vi "GetLineage.vi"(8 "error in (no error)":errorcluster, 11 "SMO in":refnum<class "SMO.lvclass">) -> (0 "error out":errorcluster, 2 "Lineage":string[](array[string]), 3 "SMO out":refnum<class "SMO.lvclass">)   [LabVIEW 2021, in "smo.lvlib" / "SMO.lvclass"]
uses:
  SMO.lvclass
  Support/Attribute.Owner/Attribute.Owner.lvclass
  SMO.lvclass/SMO.ctl
  Support/Attribute.Owner/Attribute.Owner.lvclass/Attribute.Owner.ctl
  ReftoDVR--SMO.vi
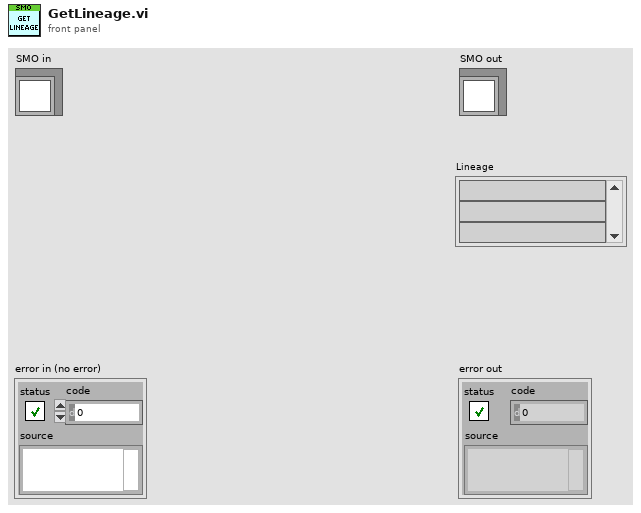
[diagram p1: front panel]
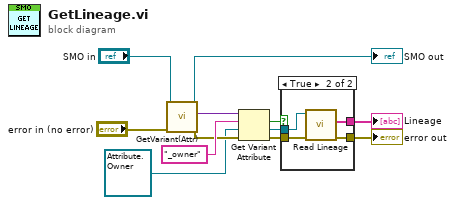
[diagram p0: block diagram]
diagram:
  n1 = call "GetVariant(Attr).vi"("error in (no error)"="error in (no error)", "SMO in"="SMO in") -> ("error out"=w7:errorcluster, "[Attributes]"=w9:variant, "SMO out"=→"SMO out":refnum<class "SMO.lvclass">)  [unwired: 7 in]
  n2 = Get Variant Attribute(Variant=w9, name="_owner", default value (empty Variant)=refnum<class "Attribute.Owner.lvclass"> refnum ("Attribute.Owner.lvclass"), error in=w7) -> (found=w1:bool, value=w4:refnum<class "Attribute.Owner.lvclass">, error out=w6:errorcluster)  [unwired: 1 out]
  n3 = case shown="True" w1 {
    tunnel: [_ w17] -> w12
    tunnel: [w13 w16] -> w11
    tunnel: w6 -> [w13 w15]
    tunnel: w4 -> [_ w14]
    frame False {
    }
    frame True {
      n4 = call "Read Lineage.vi"("error in (no error)"=w15, "Attribute.Owner in"=w14) -> ("error out"=w16:errorcluster, "Lineage"=w17:string[])  [unwired: 7 in, 1 out]
    }
  }
  "error out" <- w11
  "Lineage" <- w12
